vi "Blank URL.vi"() -> (0 "Blank URL":string)   [LabVIEW 2011]
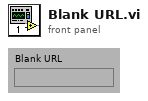
[diagram p1: front panel]
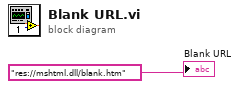
[diagram p0: block diagram]
diagram:
  "Blank URL" <- "res://mshtml.dll/blank.htm"
